vi "2014 Ball Detection.vi"(10 "Image Ctl Refnum":refnum<vi>, 11 "Src Image":T1) -> (2 "Image Out":T1(plugin-control), 3 "Ranked Objects":T5(array[cluster]) {"Score" format="%#.1g"})   [LabVIEW 2013]
uses:
  <vilib>/Rock Robotics/WPI/Camera/WPI_CameraSettings Read MJPG.ctl
  <vilib>/Rock Robotics/WPI/Camera/WPI_CameraImageSize.ctl
  <vilib>/vision/Image Controls.llb/IMAQ Image.ctl
  <vilib>/vision/NI_Vision_Development_Module.lvlib
panel:
  out "v":T1(plugin-control)
  out "s":T1(plugin-control)
  out "h":T1(plugin-control)
  in  "Std Devs":cluster{"Hue":dbl, "Sat":dbl, "Val":dbl}={"Hue"=4.0, "Sat"=6.0, "Val"=4.0}
  in  "Targets":i32=3
  in  "Area Size Limit %":dbl=0.4 format="%#_13g"
  in  "Instructions:":string="Use the tab immediately below to choose the image source. Update the camera settings or the image directory so that you have images or video to test with.\n\nCalibration:\nYou can update Color Component ranges directly, or by clicking and drawing a line across the upper third of a ball within the image -- example shown below-right.\n\nUse Debugging tab to view intermediate results. Adjust Std Dev multipliers and line to achieve the desired HSV upper and lower threshold limits.\n\nArea Size LImit is used to ignore objects too small or balls too far away to care about.\n\nTargets identifies how many of the top scores to return.\n\nThe Details tab contains center, radius, and score details of each object."
  in  "Score Cutoff":dbl(slide)=70.58823529411765 scale=0.0..100.0
  in  "Color Components":T2={"Hue"={243.23333311080933, 20.233333110809326}, "Sat"={125.60287475585938, 242.93045043945312}, "Val"={83.88507843017578, 225.38158416748047}} {"Val" scale=0.0..255.0; "Sat" scale=0.0..255.0; "Hue" scale=0.0..255.0 scale format="%#_3g"}
  out "Error":bool
  in  "Image Source":enum32{"Files", "Camera"}(tab)
  in  "List of image files":i32(listbox)
  in  "Image Directory":path=path "2014 Vision Target"
  in  "Camera Settings":T3={"fps"=15, "compression"=5, "Image Size"=enum."320x240"}
  in  "Camera IP":string="10.04.19.11"
  in  "Tabbed Info":enum32{"Debugging", "Details"}(tab)
  in  "Annotations":enum16{"None", "Good", "All"}(ring)=enum."Good"
  out "Initial Mask":T1(plugin-control)
  out "Fitted Mask":T1(plugin-control)
  # "Ranking Colors:\n1. green\n2. cyan\n3. magenta\n4. orange"
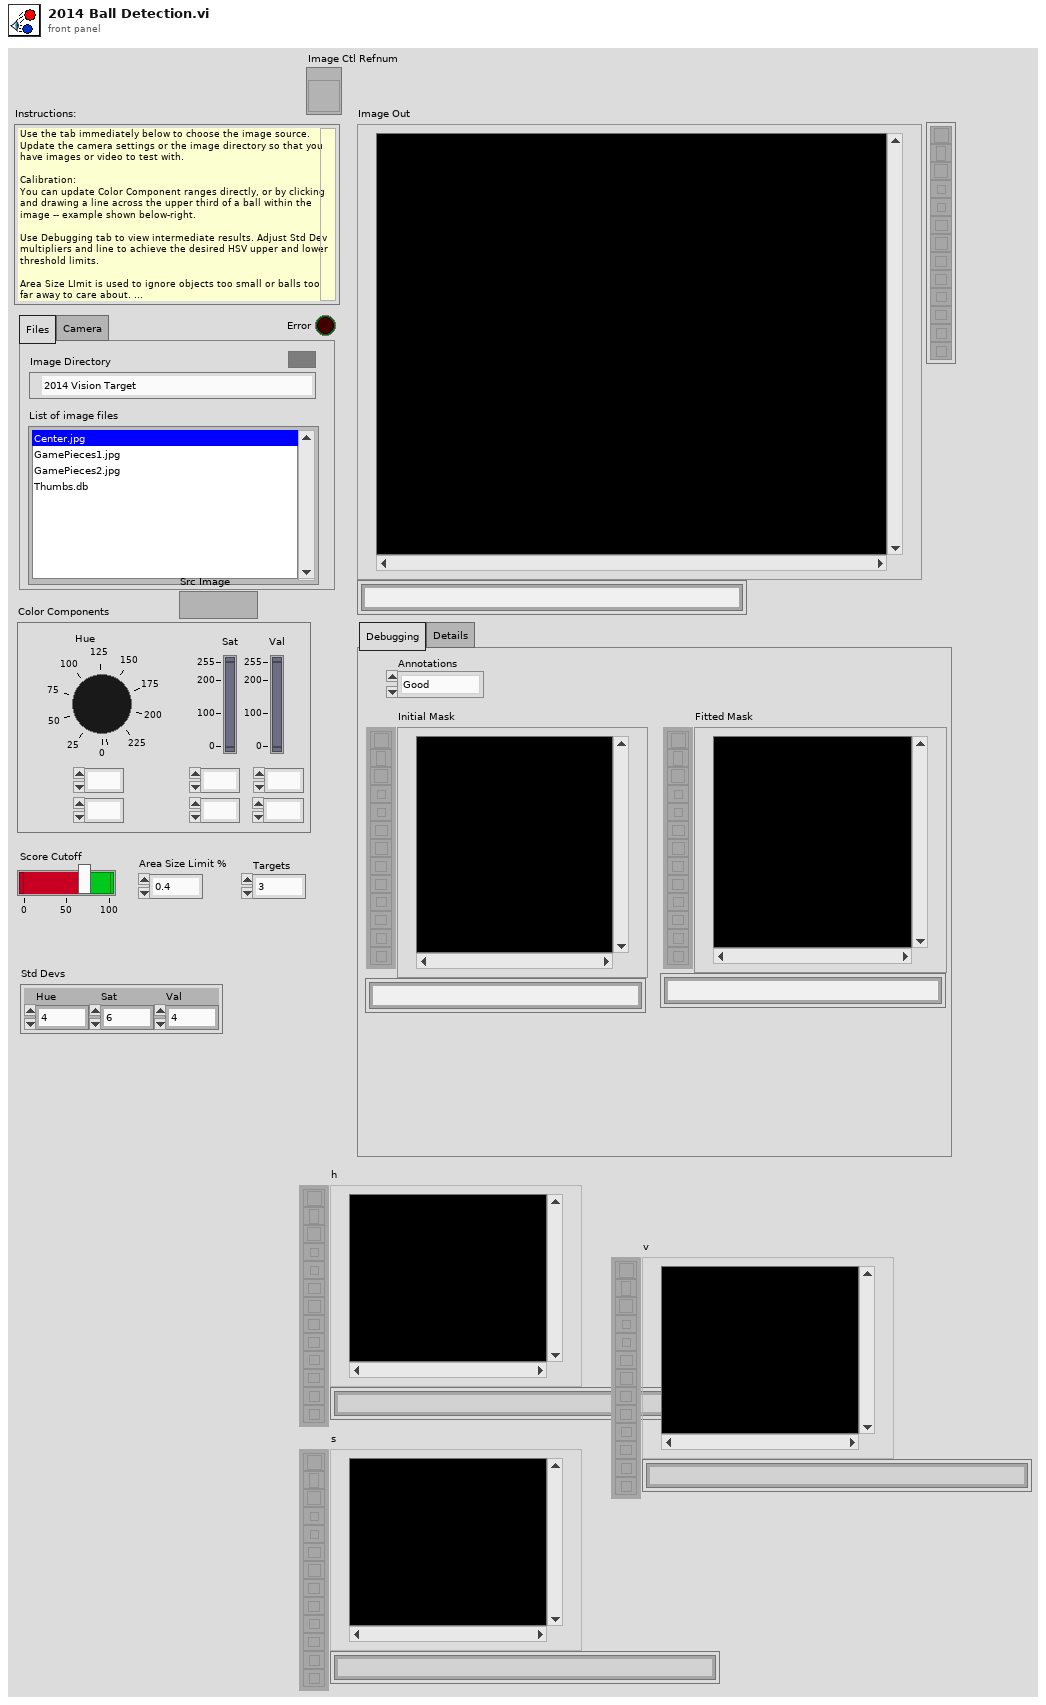
[diagram p1: front panel]
types:
  T1 = typedef "IMAQ Image.ctl" = refnum<image>
  T2 = cluster{"Hue":cluster{dbl, dbl}, "Sat":cluster{dbl, dbl}, "Val":cluster{dbl, dbl}}
  T3 = typedef "WPI_CameraSettings Read MJPG.ctl" = cluster{"fps":i32, "compression":i32, "Image Size":T4}
  T4 = typedef "WPI_CameraImageSize.ctl" = enum16{"640x480", "320x240", "160x120"}
  T5 = cluster{"Score":sgl, "Fitted Circle":cluster{"Center":cluster{"X":sgl, "Y":sgl}, "Radius":dbl, "Circle Rect":cluster{"L":sgl, "T":sgl, "R":sgl, "B":sgl}, "Roundness":dbl, "SNR (dB)":dbl}, "Search Rect":cluster{"L":sgl, "T":sgl, "R":sgl, "B":sgl}, "Details":cluster{"Edge":sgl, "Area":sgl, "Circ":sgl, "Diam":sgl}}[]
  T6 = cluster{"Circle Found":bool, "Fitted Circle":cluster{"Center":cluster{"X":sgl, "Y":sgl}, "Radius":dbl, "Center":cluster{"X":sgl, "Y":sgl}, "Radius":dbl, "Roundness":dbl, "Strength":dbl, "SNR (dB)":dbl}, "Array":dbl[], "Sorted Data":dbl[][]}[]
  T7 = cluster{"Score":dbl, "Fitted Circle":cluster{"Center (Pixels)":cluster{"X":sgl, "Y":sgl}, "Radius (Pixels)":dbl, "Circle Rect":cluster{"Left":sgl, "Top":sgl, "Right":sgl, "Bottom":sgl}, "Roundness (RW)":dbl, "Average SNR (dB)":dbl}, "Search Rect":cluster{"Left":sgl, "Top":sgl, "Right":sgl, "Bottom":sgl}, "Details":cluster{"Edges":sgl, "Circ/Rect":sgl, "Diam/Diam":sgl, "Circularity":sgl}}[]
  T8 = cluster{cluster{dbl, dbl}, cluster{dbl, dbl}, cluster{dbl, dbl}}
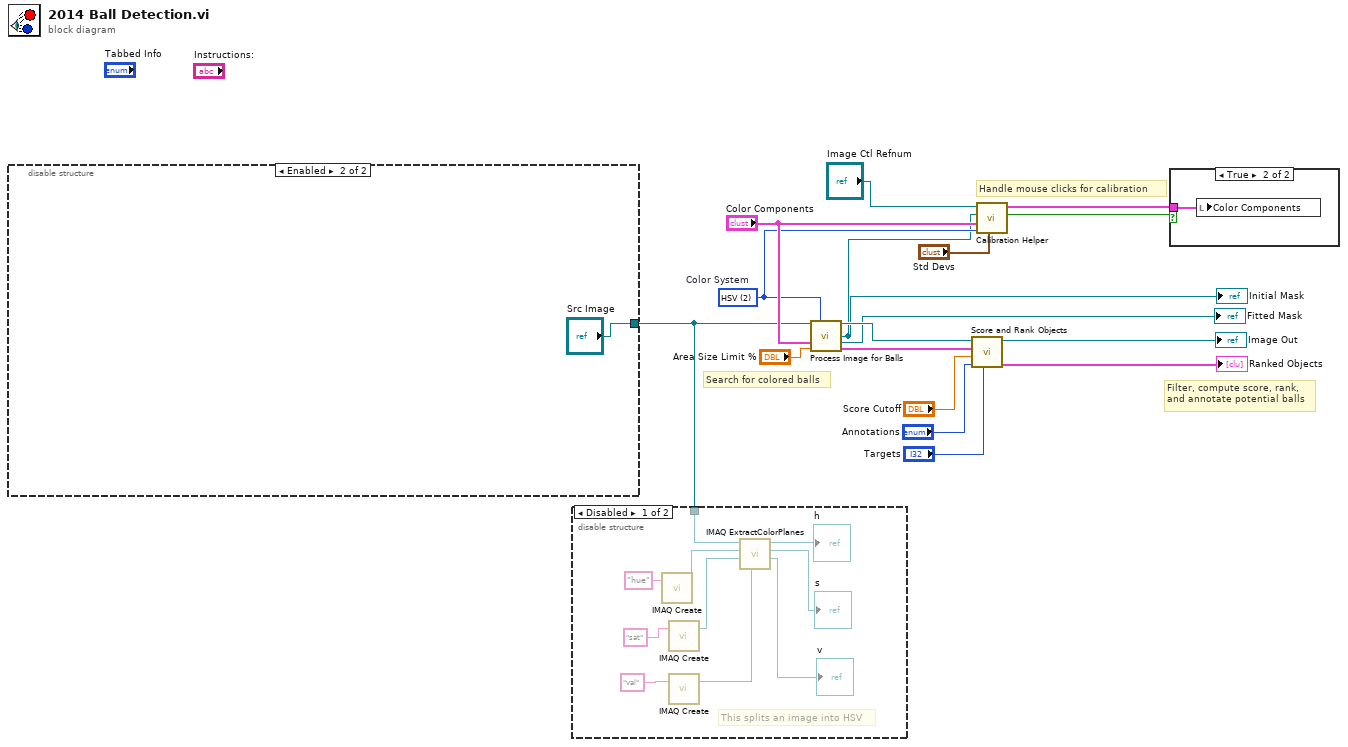
[diagram p0: block diagram]
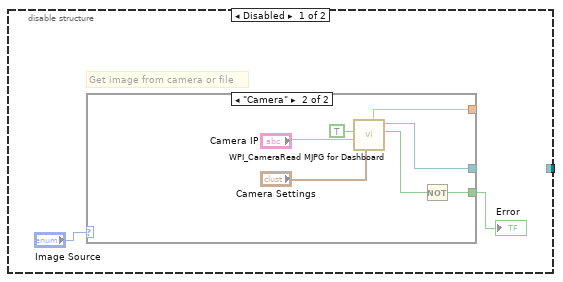
[diagram p3: hidden frame]
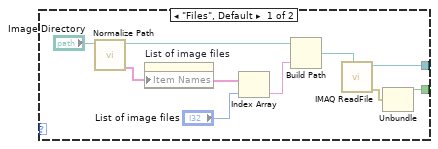
[diagram p4: hidden frame]
diagram:
  w7 = u16 2 items=["RGB", "HSL", "HSV", "HSI"]  # Color System
  # "Search for colored balls"
  # "Handle mouse clicks for calibration"
  # "Filter, compute score, rank,\nand annotate potential balls"
  n1 = disable-structure shown="Enabled" {
    disable-tunnel: [_ "Src Image"] -> w1
    frame Disabled {
      # "Get image from camera or file"
      n2 = case shown="\"Camera\"" "Image Source" {
        tunnel: [w25 w35] -> _
        tunnel: [w23 w30] -> w18
        tunnel: [_ w29] -> _
        frame "Files", Default {
          n3 = call "Normalize Path.vi"("Image Directory"="Image Directory") -> ("Filenames"=w22:string[], "Path"=w20:path)  [unwired: 9 in]
          n4 = property on="List of image files" class="LstBox (strict)"("Item Names"=w22) -> ()  [unwired: 2 in, 2 out]
          n5 = Index Array(array=w22, index="List of image files") -> (element=w27:string)
          n6 = Build Path(base path=w20, name or relative path=w27) -> (appended path=w26:path)
          n7 = call "IMAQ ReadFile"("File Path"=w26) -> ("error out"=w24:errorcluster, "Image Out"=w25:T1)  [unwired: 6 in, 3 out]
          n8 = Unbundle(w24) -> ("status"=w23:bool)  [unwired: 2 out]
        }
        frame "Camera" {
          n9 = call <vilib>:"WPI_CameraRead MJPG for Dashboard.vi"("Camera Settings"="Camera Settings", "Camera IP"="Camera IP", "Enable"=TRUE) -> ("Active"=w32:bool, "Refnum out"=w35:T1, "Bandwidth (Mbps)"=w29:dbl)  [unwired: 5 in, 1 out]
          n10 = Not(x=w32) -> (.not. x?=w30:bool)
        }
      }
      "Error" <- w18
    }
    frame Enabled {
    }
  }
  n11 = disable-structure shown="Disabled" {
    disable-tunnel: w1 -> [w46 _]
    frame Disabled {
      # "This splits an image into HSV"
      n12 = call "IMAQ Create"("Image Name"="hue") -> ("New Image"=w42:T1)  [unwired: 4 in, 1 out]
      n13 = call "IMAQ Create"("Image Name"="sat") -> ("New Image"=w41:T1)  [unwired: 4 in, 1 out]
      n14 = call "IMAQ Create"("Image Name"="val") -> ("New Image"=w40:T1)  [unwired: 4 in, 1 out]
      n15 = call "IMAQ ExtractColorPlanes"("Blue or Luma or Val or Inten Plane"=w40, "Green or Sat Plane"=w41, "Red or Hue Plane"=w42, "Image Src"=w46) -> ("Blue or Luma or Val or Inten Plane out"=→"v":T1, "Green or Sat Plane out"=→"s":T1, "Red or Hue Plane out"=→"h":T1)  [unwired: 4 in, 1 out]
    }
    frame Enabled {
    }
  }
  n16 = call "Process Image for Balls.vi"("Src Image"=w1, "Color Mode 2"=w7, "Color"="Color Components", "Area Cutoff %"="Area Size Limit %") -> ("Src Image Out"=w13:T1, "First Threshold"=w5:T1, "Fitted"=→"Fitted Mask":T1, "Potential"=w12:T6)  [unwired: 8 in]
  "Initial Mask" <- w5
  n17 = call "Score and Rank Objects.vi"("Targets"="Targets", "Annotations"="Annotations", "Score Limit"="Score Cutoff", "Object Info"=w12, "Image in"=w13) -> ("Object Info"=→"Ranked Objects":T7, "Annotated Image"=→"Image Out":T1)  [unwired: 5 in]
  n18 = call "Calibration Helper.vi"("Std Devs"="Std Devs", "Color Mode"=w7, "Color Components"="Color Components", "Image"=w5, "Image Ctl Refnum"="Image Ctl Refnum") -> ("Changed"=w3:bool, "output color"=w4:T8)  [unwired: 5 in]
  n19 = case shown="True" w3 {
    tunnel: w4 -> [_ w47]
    frame False {
    }
    frame True {
      n20 = local write "Color Components"(w47) -> ()
    }
  }
